vi "file -- scan filename logic -- datestring.vi"(7 "scan filename action":T1, 8 "time stamp IN":timestamp=timestamp(19856294.882018566 s since 1904-01-01), 11 "date/time string IN":string) -> (0 "time stamp OUT":timestamp, 1 "parse OK":bool, 2 "date string regexp":string, 3 "date/time string OUT":string)   [LabVIEW 2016]
uses:
  resonant_ultrasound/maglab ultrasound -- arkady/file -- scan filename action.ctl
  <vilib>/Utility/miscctls.llb/LVDateTimeRec.ctl
  resonant_ultrasound/maglab ultrasound -- arkady/Q - not nan -- integer.vi
  <vilib>/regexp/Match Regular Expression.xnode
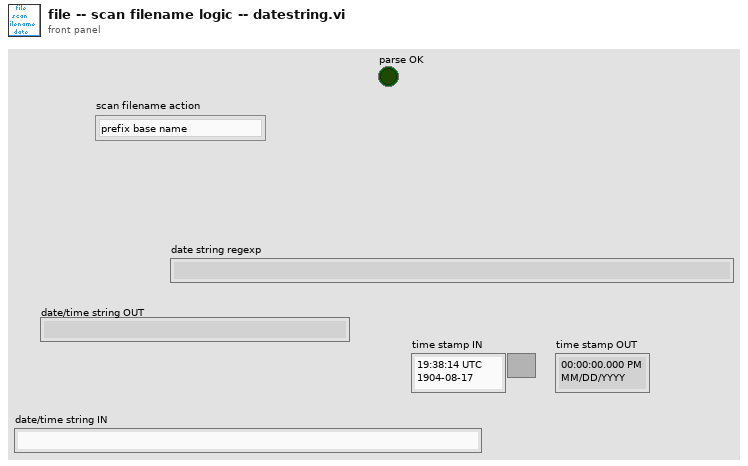
[diagram p1: front panel]
types:
  T1 = typedef "file -- scan filename action.ctl" = enum16{"prefix base name", "datestring regexp", "parse datestring", "datestring", "filename regexp", "parse filename", "datestring regexp (no brackets)", "suffix base name"}
  T2 = typedef "LVDateTimeRec.ctl" = cluster{"fractional second":dbl, "second":i32, "minute":i32, "hour":i32, "day of month":i32, "month":i32, "year":i32, "day of week":i32, "day of year":i32, "DST":i32}
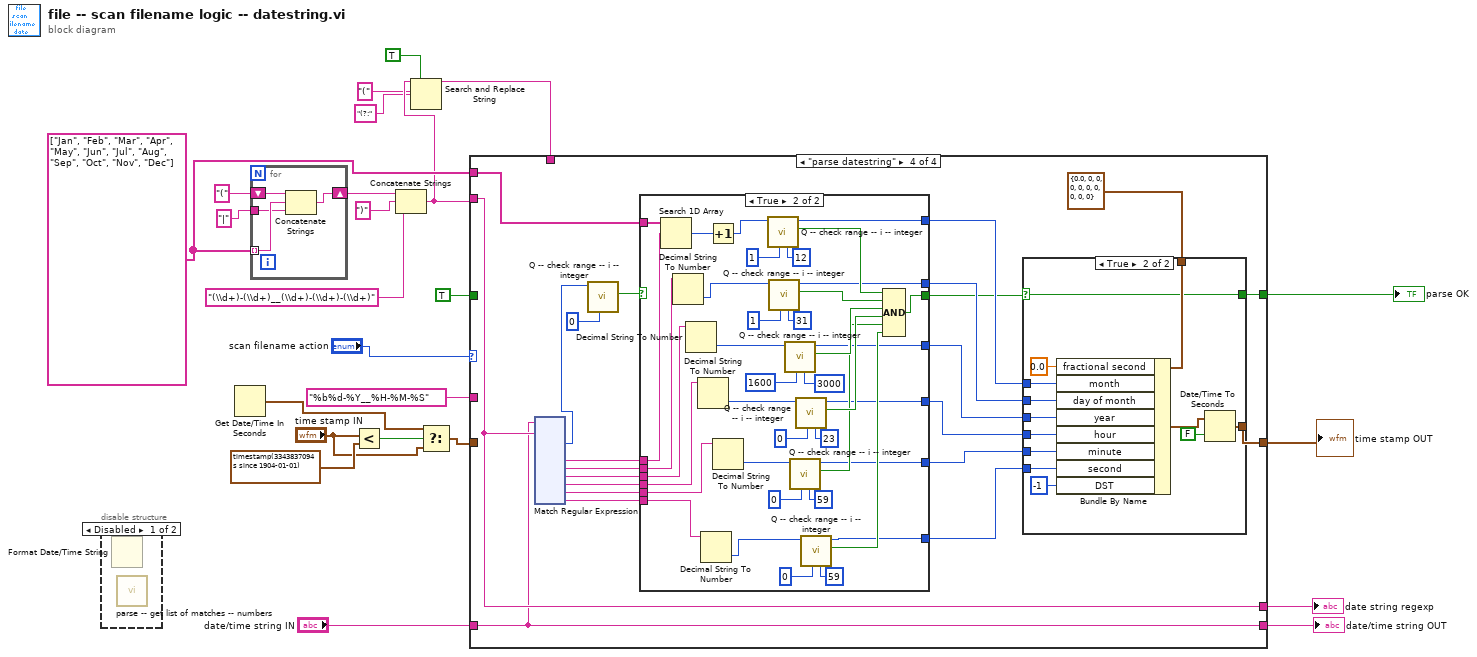
[diagram p0: block diagram]
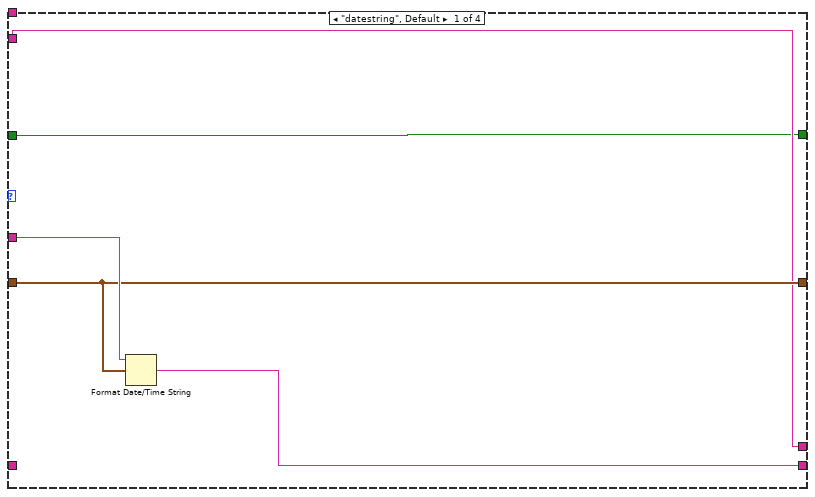
[diagram p3: hidden frame]
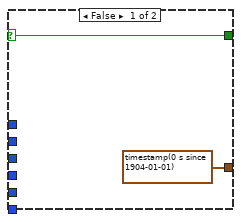
[diagram p6: hidden frame]
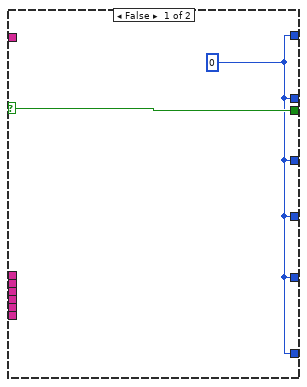
[diagram p7: hidden frame]
diagram:
  w15 = string[] ["Jan", "Feb", "Mar", "Apr", "May", "Jun", "Jul", "Aug", "Sep", "Oct", "Nov", "Dec"]
  n1 = disable-structure shown="Disabled" {
    frame Disabled {
      n2 = Format Date/Time String() -> ()  [unwired: 3 in, 1 out]
      n3 = call "parse -- get list of matches -- numbers.vi"() -> ()  [unwired: 8 in, 4 out]
    }
    frame Enabled {
    }
  }
  n4 = Get Date/Time In Seconds() -> (seconds since 1Jan1904=w9:timestamp)
  n5 = for {
    shift-right: [w28] -> w20
    shift-left: "(" ("time format string (%c)") -> [w27]
    tunnel: w15 -> [w26] mode=indexing
    tunnel: "|" ("time format string (%c)") -> [w25]
    n6 = Concatenate Strings(w27, w26, w25) -> (w28:string)
  }
  n7 = Less?(x="time stamp IN", y=timestamp(3343837094.8820186 s since 1904-01-01) ("current time")) -> (x < y?=w10:bool)
  n8 = Concatenate Strings(w20, ")" ("time format string (%c)"), "(\\d+)-(\\d+)__(\\d+)-(\\d+)-(\\d+)" ("time format string (%c)")) -> (w5:string)
  n9 = Search and Replace String(replace all?=TRUE ("replace all? (F)"), input string=w5, search string="(" ("time format string (%c)"), replace string="(?:" ("time format string (%c)")) -> (result string=w2:string)  [unwired: 4 in, 3 out]
  n10 = Select(t=w9, s=w10, f="time stamp IN") -> (s? t:f=w8:timestamp)
  n11 = case shown="\"parse datestring\"" "scan filename action" {
    tunnel: w8 -> [w31 w35 w40 _]
    tunnel: "%b%d-%Y__%H-%M-%S" ("time format string (%c)") -> [w33 _ _ _]
    tunnel: [w32 w36 w41 w62] -> w23
    tunnel: [w30 w37 w38 w63] -> w17
    tunnel: w5 -> [w30 w37 _ w63]
    tunnel: "date/time string IN" -> [_ w36 w41 w62]
    tunnel: w15 -> [_ _ _ w61]
    tunnel: [w31 w35 w40 w51] -> w14
    tunnel: [w29 w34 w39 w42] -> w13
    tunnel: TRUE -> [w29 w34 w39 _]
    tunnel: w2 -> [_ _ w38 _]
    frame "datestring", Default {
      n12 = Format Date/Time String(time format string (%c)=w33, seconds (now)=w31) -> (date/time string=w32:string)  [unwired: 1 in]
    }
    frame "datestring regexp" {
    }
    frame "datestring regexp (no brackets)" {
    }
    frame "parse datestring" {
      n13 = xnode "Match Regular Expression"("input string"=w62, "regular expression"=w63) -> ("offset past match"=w53:i32, "submatch 1"=w60:string, "submatch 2"=w59:string, "submatch 3"=w58:string, "submatch 4"=w57:string, "submatch 5"=w56:string, "submatch 6"=w55:string)  [unwired: 4 in, 4 out]
      n14 = call "Q -- check range -- i -- integer.vi"("lower"=0, "number"=w53) -> ("in range?"=w52:bool)  [unwired: 7 in, 2 out]
      n15 = case shown="True" w52 {
        selector: w52 -> [w80 _]
        tunnel: w61 -> [_ w119]
        tunnel: w60 -> [_ w118]
        tunnel: w59 -> [_ w117]
        tunnel: w58 -> [_ w116]
        tunnel: w57 -> [_ w115]
        tunnel: w56 -> [_ w114]
        tunnel: w55 -> [_ w113]
        tunnel: [w80 w89] -> w43
        tunnel: [w79 w88] -> w49
        tunnel: [w79 w87] -> w48
        tunnel: [w79 w86] -> w47
        tunnel: [w79 w85] -> w46
        tunnel: [w79 w84] -> w45
        tunnel: [w79 w83] -> w44
        frame False {
          w79 = 0 ("number in range")
        }
        frame True {
          n16 = Search 1D Array(1D array=w119, element=w118) -> (index of element=w112:i32)  [unwired: 1 in]
          n17 = Decimal String To Number(string=w117) -> (number=w82:i32)  [unwired: 2 in, 1 out]
          n18 = Decimal String To Number(string=w116) -> (number=w98:i32)  [unwired: 2 in, 1 out]
          n19 = Decimal String To Number(string=w115) -> (number=w97:i32)  [unwired: 2 in, 1 out]
          n20 = Decimal String To Number(string=w113) -> (number=w81:i32)  [unwired: 2 in, 1 out]
          n21 = Increment(x=w112) -> (x+1=w111:i32)
          n22 = Decimal String To Number(string=w114) -> (number=w96:i32)  [unwired: 2 in, 1 out]
          n23 = call "Q -- check range -- i -- integer.vi"("upper"=12, "lower"=1, "number"=w111) -> ("in range?"=w95:bool, "number in range"=w88:i32)  [unwired: 6 in, 1 out]
          n24 = call "Q -- check range -- i -- integer.vi"("upper"=31, "lower"=1, "number"=w82) -> ("in range?"=w94:bool, "number in range"=w83:i32)  [unwired: 6 in, 1 out]
          n25 = call "Q -- check range -- i -- integer.vi"("upper"=3000, "lower"=1600, "number"=w98) -> ("in range?"=w93:bool, "number in range"=w84:i32)  [unwired: 6 in, 1 out]
          n26 = call "Q -- check range -- i -- integer.vi"("upper"=59, "lower"=0, "number"=w96) -> ("in range?"=w91:bool, "number in range"=w86:i32)  [unwired: 6 in, 1 out]
          n27 = call "Q -- check range -- i -- integer.vi"("upper"=23, "lower"=0, "number"=w97) -> ("in range?"=w92:bool, "number in range"=w85:i32)  [unwired: 6 in, 1 out]
          n28 = call "Q -- check range -- i -- integer.vi"("upper"=59, "lower"=0, "number"=w81) -> ("in range?"=w90:bool, "number in range"=w87:i32)  [unwired: 6 in, 1 out]
          n29 = Compound Arithmetic op=AND(w95, w94, w93, w92, w91, w90) -> (w89:bool)
        }
      }
      n30 = case shown="True" w43 {
        selector: w43 -> [w64 w68]
        tunnel: [timestamp(0 s since 1904-01-01) ("time stamp") w78] -> w51
        tunnel: T2 {"fractional second"=0.0, "second"=0, "minute"=0, "hour"=0, "day of month"=0, "month"=0, "year"=0, "day of week"=0, "day of year"=0, "DST"=0} ("date time rec") -> [_ w77]
        tunnel: w49 -> [_ w76]
        tunnel: w48 -> [_ w74]
        tunnel: w47 -> [_ w73]
        tunnel: w46 -> [_ w72]
        tunnel: w45 -> [_ w71]
        tunnel: w44 -> [_ w70]
        tunnel: [w64 w68] -> w42
        frame False {
        }
        frame True {
          n31 = Bundle By Name(cluster=w77, "fractional second"=0.0, "month"=w76, "day of month"=w70, "year"=w71, "hour"=w72, "minute"=w73, "second"=w74, "DST"=-1) -> (w69:T2)
          n32 = Date/Time To Seconds(1:FALSE ("is UTC (F)"), 2:w69) -> (0:w78:timestamp)
        }
      }
    }
  }
  "date/time string OUT" <- w23
  "date string regexp" <- w17
  "time stamp OUT" <- w14
  "parse OK" <- w13
